vi "Measure Digital Pulse Width (mSec).vi"(7 "cycles to filter (0)":u16, 9 "inverted pulse (F)":bool, 10 "timeout (mSec)":i32=18, 11 "FPGA digital input":refnum<k21>="Port0/DIO0") -> (1 "timed out?":bool, 3 "pulse width (mSec)":u32)   [LabVIEW 2017, in "NI_Robotics_FPGA Utilities.lvlib"]
uses:
  <vilib>/robotics/Utilities/FPGA Utilities/NI_Robotics_FPGA Utilities.lvlib
  <vilib>/Platform/TimedLoop/XDataNode/XDataNode.xnode
  <vilib>/Platform/TimedLoop/XDataNode/nitl_modes.ctl
  <vilib>/Platform/TimedLoop/XDataNode/XDNodeRunTimeDep.lvlib
  <vilib>/Platform/TimedLoop/XDataNode/wakeup.ctl
  <vilib>/Platform/TimedLoop/XDataNode/timing_clust.ctl
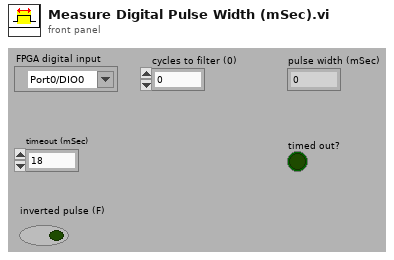
[diagram p1: front panel]
types:
  T1 = typedef "XDNodeRunTimeDep.lvlib/timing_clust.ctl" = cluster{"Expected End [f-1]":u64, "Actual End [f-1]":u64, "Finished Late? [f-1]":bool, "Expected End [i-1]":u64, "Actual End [i-1]":u64, "Finished Late? [i-1]":bool, "Expected Start [i]":u64, "Actual Start [i]":u64, "Expected Start [f]":u64, "Actual Start [f]":u64, "Source Name":string, "Structure Name":string, "Period":i64, "Deadline":i64, "Offset":i64, "Start":i64, "Priority":i32, "Timeout":i32, "Mode":T2, "Wakeup Reason":T3, "Error":errorcluster, "Source Type":string, "Secondary Source Type":string, "Global End Time":u64, "Global Start Time":u64, "Frame Duration":u64, "Iteration Duration":u64, "Assigned CPU":i32, "I/O Scan Engine Mode":u32}
  T2 = typedef "XDNodeRunTimeDep.lvlib/nitl_modes.ctl" = enum32{"No Change", "Process missed periods, maintain original phase", "Discard missed periods, maintain original phase", "Process missed periods, ignore original phase", "Discard missed periods, ignore original phase"}
  T3 = typedef "XDNodeRunTimeDep.lvlib/wakeup.ctl" = enum32{"Normal", "Aborted", "Asynchronous wakeup", "Timing source error", "Timed loop error", "Timeout"}
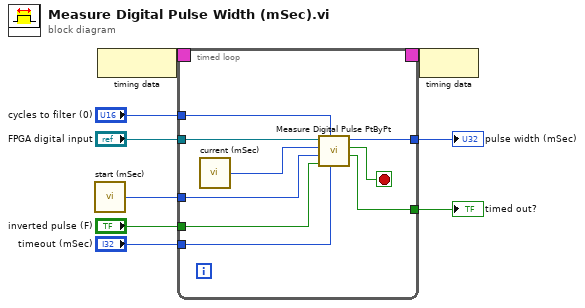
[diagram p0: block diagram]
diagram:
  n1 = call "start (mSec)"() -> ("Tick Count(mSec)"=w1:u32)
  n2 = node-c288() -> (w9:T1)
  n3 = timed-loop {
    timing: w9 -> [_]
    timing-out: [_] -> w8
    tunnel: "FPGA digital input" -> [w18]
    tunnel: "timeout (mSec)" -> [w12]
    tunnel: "inverted pulse (F)" -> [w17]
    tunnel: [w15] -> w4
    tunnel: [w14] -> w3
    tunnel: "cycles to filter (0)" -> [w13]
    tunnel: w1 -> [w10]
    stop <- w16 stop-if-true
    n4 = call "current (mSec)"() -> ("Tick Count(mSec)"=w11:u32)
    n5 = call <vilib>:"Measure Digital Pulse PtByPt.vi"("timeout (units)"=w12, "cycles to filter (0)"=w13, "inverted pulse (F)"=w17, "start time (units)"=w10, "current time (units)"=w11, "FPGA digital input"=w18) -> ("timed out?"=w15:bool, "stopped?"=w16:bool, "pulse width (units)"=w14:u32)  [unwired: 3 in]
  }
  "timed out?" <- w4
  "pulse width (mSec)" <- w3
  n6 = node-c288(w8) -> ()
